vi "ASCII 쓰기.vi"() -> ()   [LabVIEW 2014]
panel:
  in  "텍스트":string
  out "에러 출력":errorcluster
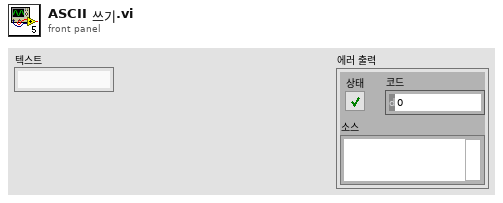
[diagram p1: front panel]
types:
  T1 = enum16{"open", "replace", "create", "open or create", "replace or create", "replace or create with confirmation"}
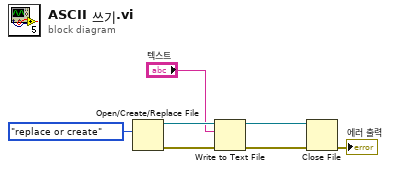
[diagram p0: block diagram]
diagram:
  n1 = Open/Create/Replace File(operation (0:open)=T1."replace or create" ("동작(0:open)")) -> (refnum out=w6:refnum<file>, error out=w4:errorcluster)  [unwired: 5 in, 1 out]
  n2 = Write to Text File(file (use dialog)=w6, text="텍스트", error in=w4) -> (refnum out=w5:refnum<file>, error out=w3:errorcluster)  [unwired: 1 in, 1 out]
  n3 = Close File(refnum=w5, error in=w3) -> (error out=→"에러 출력":errorcluster)  [unwired: 1 out]
